vi "add-dll.vi"(8 "y":dbl, 9 "x":dbl) -> (3 "x+y":dbl)   [LabVIEW 2018]
panel:
  # "INPUT"
  # "OUTPUT"
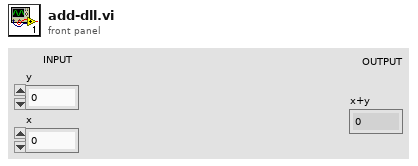
[diagram p1: front panel]
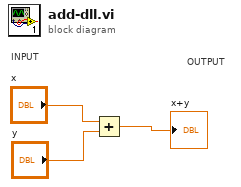
[diagram p0: block diagram]
diagram:
  # "OUTPUT"
  # "INPUT"
  n1 = Add(x="x", y="y") -> (x+y=→"x+y":dbl)
